vi "GetParam.vi"(8 "error in (no error)":errorcluster caption="entrée d'erreur (pas d'erreur)", 11 "Olivetti_faces.lvclass":refnum<class "Olivetti_faces.lvclass">) -> (0 "error out":errorcluster caption="sortie d'erreur", 2 "fetch_olivetti_faces":T1={"shuffle"=FALSE, "random_state"=0, "download_if_missing"=TRUE, "Returns"="Data"} {"random_state" min=-1}, 3 "Olivetti_faces.lvclass":refnum<class "Olivetti_faces.lvclass">)   [LabVIEW 2020, in "Olivetti_faces.lvclass"]
doc: "Get parameters"
uses:
  Olivetti_faces.lvclass
  Olivetti_faces.lvclass/Olivetti_faces.ctl
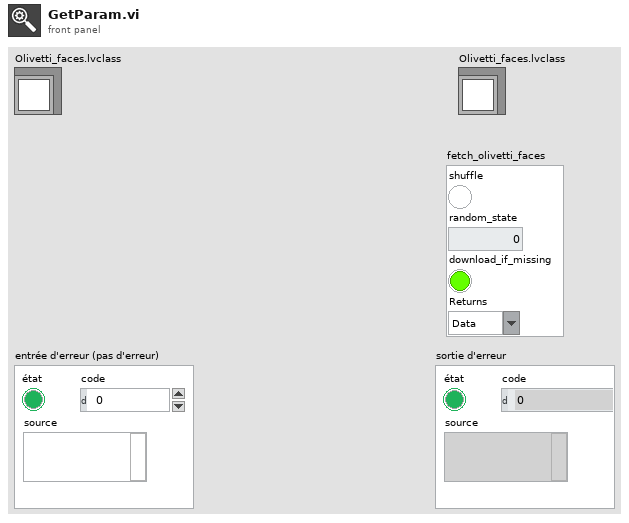
[diagram p1: front panel]
types:
  T1 = cluster{"shuffle":bool, "random_state":i32, "download_if_missing":bool, "Returns":string}
  T2 = cluster{"shuffle":bool, "random_state":i32, " download_if_missing ":bool, "Returns":string}
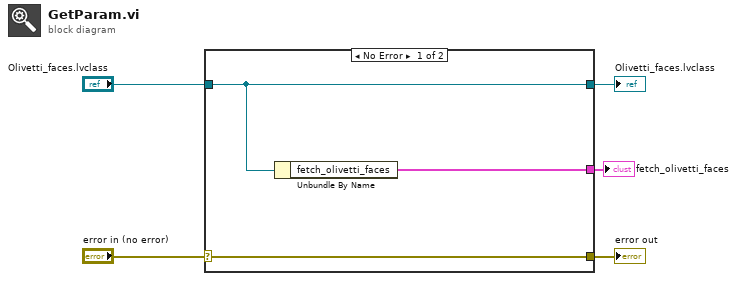
[diagram p0: block diagram]
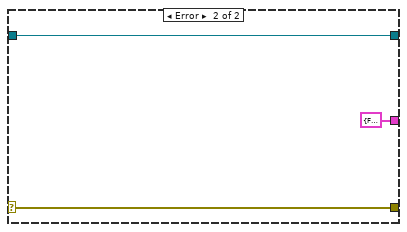
[diagram p2: hidden frame]
diagram:
  n1 = case shown="No Error" "error in (no error)" {
    selector: "error in (no error)" -> [w8 w10]
    tunnel: [w8 w10] -> w4
    tunnel: [w6 w11] -> w2
    tunnel: "Olivetti_faces.lvclass" -> [w6 w11]
    tunnel: [w7 T2 {"shuffle"=FALSE, "random_state"=0, " download_if_missing "=FALSE, "Returns"=""} ("fetch_olivetti_faces")] -> w1
    frame No Error {
      n2 = Unbundle By Name(w6) -> ("fetch_olivetti_faces"=w7:T2)
    }
    frame Error {
    }
  }
  "error out" <- w4
  "Olivetti_faces.lvclass" <- w2
  "fetch_olivetti_faces" <- w1
